vi "Get JSON Data.vi"(7 "Panel Origin":T1, 8 "error in (no error)":errorcluster, 9 "Force Get All Data":bool, 10 "VI Reference":refnum<vi>, 11 "Select In":refnum<class "Select.lvclass">) -> (0 "error out":errorcluster, 2 "JSON string":string, 3 "Select Out":refnum<class "Select.lvclass">)   [LabVIEW 2015, in "Front Panel Publisher.lvlib" / "Select.lvclass"]
uses:
  Select.lvclass
  <vilib>/Utility/miscctls.llb/LVPointTypeDef.ctl
  Text_class/Text.lvclass
  Control_class/Control.lvclass
  Object_class/Object.lvclass
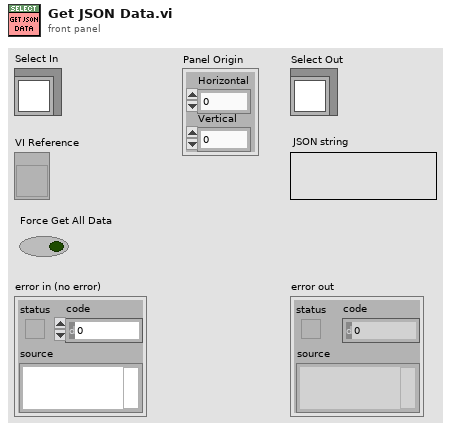
[diagram p1: front panel]
types:
  T1 = typedef "LVPointTypeDef.ctl" = cluster{"Horizontal":i16, "Vertical":i16}
  T2 = typedef "Front Panel Publisher.lvlib/Object.lvclass/Attributes.ctl" = cluster{"UID":i32, "Type":string, "Coordinates":T3, "Reference":refnum<vi>}
  T3 = typedef "Front Panel Publisher.lvlib/Object.lvclass/Coordinates.ctl" = cluster{"Left":i32, "Top":i32, "Height":u32, "Width":u32}
  T4 = typedef "Front Panel Publisher.lvlib/Control.lvclass/Attributes.ctl" = cluster{"Description":string, "Indicator":bool, "Default Value":variant, "Control Index":i32, "Label":refnum<class "Text.lvclass">, "Caption":refnum<class "Text.lvclass">, "Image b64":string, "Use Picture":bool, "Value Only":bool}
  T5 = typedef "Front Panel Publisher.lvlib/Select.lvclass/Attributes.ctl" = cluster{"Ring Image Variable Name":string}
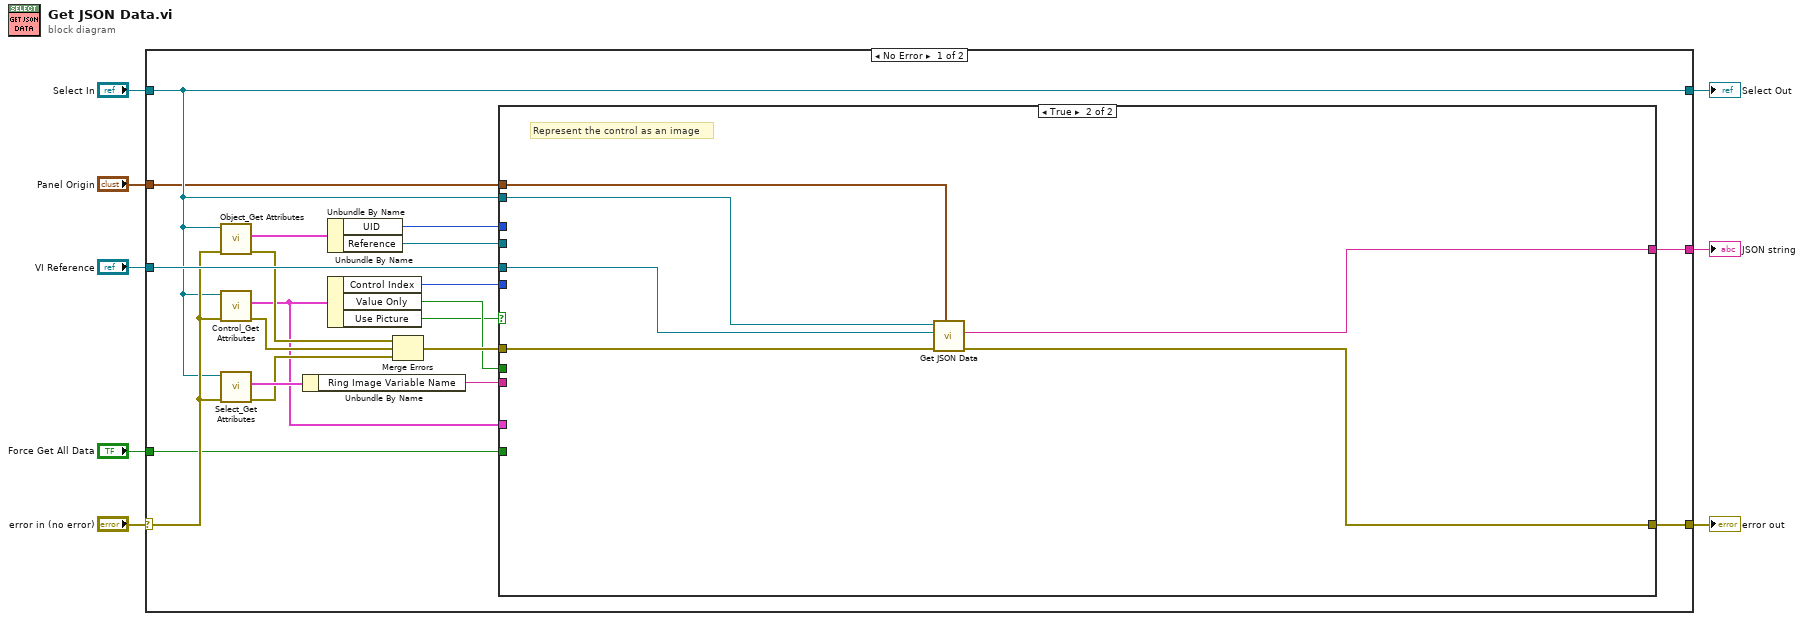
[diagram p0: block diagram]
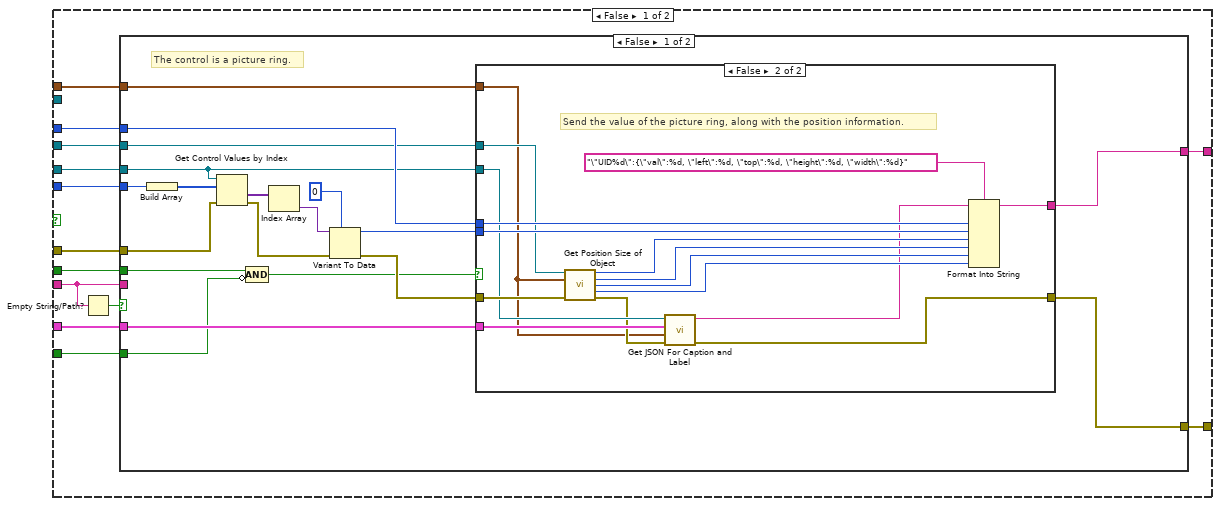
[diagram p2: hidden frame]
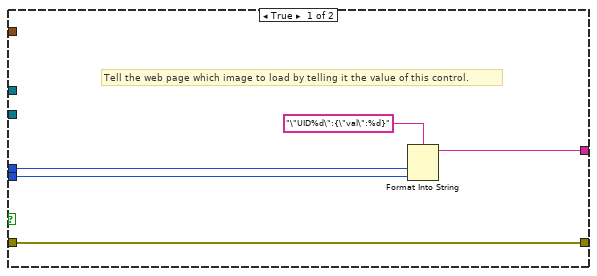
[diagram p3: hidden frame]
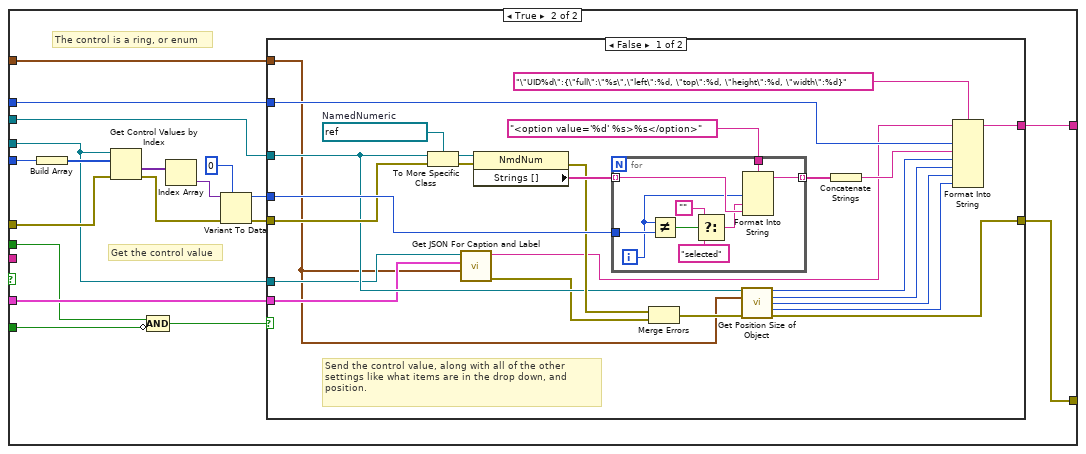
[diagram p4: hidden frame]
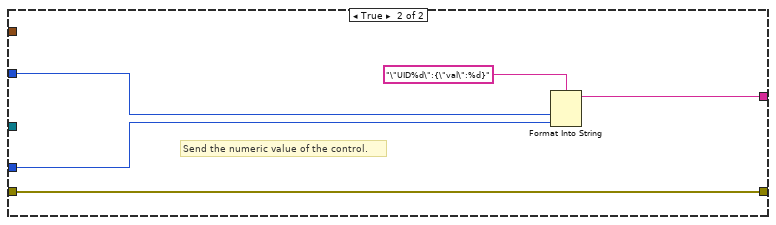
[diagram p5: hidden frame]
diagram:
  n1 = case shown="No Error" "error in (no error)" {
    selector: "error in (no error)" -> [w19 w147]
    tunnel: [w27 w147] -> w7
    tunnel: [w12 w146] -> w5
    tunnel: "Select In" -> [w12 w146]
    tunnel: "VI Reference" -> [w25 _]
    tunnel: [w24 _] -> w3
    tunnel: "Force Get All Data" -> [w10 _]
    tunnel: "Panel Origin" -> [w9 _]
    frame No Error {
      n2 = call "Object_Get Attributes.vi"("error in (no error)"=w19, "Object In"=w12) -> ("error out"=w17:errorcluster, "Data"=w23:T2)  [unwired: 6 in, 2 out]
      n3 = call "Control_Get Attributes.vi"("error in (no error)"=w19, "Control In"=w12) -> ("error out"=w28:errorcluster, "Data"=w11:T4)  [unwired: 6 in, 2 out]
      n4 = call "Select_Get Attributes.vi"("error in (no error)"=w19, "Select In"=w12) -> ("error out"=w16:errorcluster, "Data"=w20:T5)  [unwired: 6 in, 2 out]
      n5 = Unbundle By Name(w20) -> ("Ring Image Variable Name"=w15:string)
      n6 = Unbundle By Name(w23) -> ("UID"=w22:i32, "Reference"=w21:refnum<vi>)
      n7 = Unbundle By Name(w11) -> ("Control Index"=w26:i32, "Value Only"=w14:bool, "Use Picture"=w13:bool)
      n8 = Merge Errors(w17, w28, w16) -> (w18:errorcluster)
      n9 = case shown="True" w13 {
        tunnel: [w41 w142] -> w27
        tunnel: w26 -> [w40 _]
        tunnel: w25 -> [w39 w144]
        tunnel: [w38 w141] -> w24
        tunnel: w22 -> [w37 _]
        tunnel: w21 -> [w36 _]
        tunnel: w18 -> [w35 w143]
        tunnel: w15 -> [w33 _]
        tunnel: w14 -> [w32 _]
        tunnel: w12 -> [_ w145]
        tunnel: w11 -> [w31 _]
        tunnel: w10 -> [w30 _]
        tunnel: w9 -> [w29 w140]
        frame False {
          n10 = Empty String/Path?(string/path=w33) -> (empty?=w34:bool)
          n11 = case shown="False" w34 {
            tunnel: [w48 w100] -> w41
            tunnel: w40 -> [w55 w99]
            tunnel: w39 -> [w46 w87]
            tunnel: [w53 w98] -> w38
            tunnel: w37 -> [w54 w97]
            tunnel: w36 -> [w50 w88]
            tunnel: w35 -> [w52 w96]
            tunnel: w33 -> [_ _]
            tunnel: w32 -> [w44 w84]
            tunnel: w31 -> [w47 w86]
            tunnel: w30 -> [w45 w85]
            tunnel: w29 -> [w42 w82]
            frame False {
              # "The control is a picture ring."
              n12 = Build Array(w55) -> (w59:i32[])
              n13 = Get Control Values by Index(0:w46, 1:w59, 3:w52) -> (10:w58:variant[], 11:w60:errorcluster)
              n14 = Compound Arithmetic op=AND(w44, invert w45) -> (w43:bool)
              n15 = Index Array(array=w58) -> (element=w57:variant)  [unwired: 1 in]
              n16 = Variant To Data(error in=w60, type=0, Variant=w57) -> (data=w51:i32, error out=w49:errorcluster)
              n17 = case shown="False" w43 {
                tunnel: w54 -> [w65 w81]
                tunnel: [w64 w80] -> w53
                tunnel: w51 -> [w63 w79]
                tunnel: w50 -> [_ w77]
                tunnel: w49 -> [w61 w72]
                tunnel: [w61 w67] -> w48
                tunnel: w47 -> [_ w71]
                tunnel: w46 -> [_ w70]
                tunnel: w42 -> [_ w66]
                frame True {
                  # "Tell the web page which image to load by telling it the value of this control."
                  n18 = Format Into String(format string="\"UID%d\":{\"val\":%d}", w65, w63) -> (resulting string=w64:string)  [unwired: 2 in, 1 out]
                }
                frame False {
                  # "Send the value of the picture ring, along with the position information."
                  n19 = call "Get Position Size of Object.vi"("GObject in"=w77, "Panel Origin"=w66, "error in (no error)"=w72) -> ("Left"=w76:i32, "Top"=w75:i32, "Height"=w74:u32, "Width"=w73:u32, "error out"=w68:errorcluster)  [unwired: 8 in]
                  n20 = call "Get JSON For Caption and Label.vi"("error in (no error)"=w68, "Panel Origin"=w66, "Data"=w71, "VI in"=w70) -> ("error out"=w67:errorcluster, "JSON"=w69:string)  [unwired: 6 in]
                  n21 = Format Into String(format string="\"UID%d\":{\"val\":%d, \"left\":%d, \"top\":%d, \"height\":%d, \"width\":%d}", initial string=w69, w81, w79, w76, w75, w74, w73) -> (resulting string=w80:string)  [unwired: 1 in, 1 out]
                }
              }
            }
            frame True {
              # "Get the control value"
              # "The control is a ring, or enum"
              n22 = Build Array(w99) -> (w93:i32[])
              n23 = Get Control Values by Index(0:w87, 1:w93, 3:w96) -> (10:w92:variant[], 11:w95:errorcluster)
              n24 = Compound Arithmetic op=AND(w84, invert w85) -> (w83:bool)
              n25 = Index Array(array=w92) -> (element=w91:variant)  [unwired: 1 in]
              n26 = Variant To Data(error in=w95, type=0, Variant=w91) -> (data=w89:i32, error out=w94:errorcluster)
              n27 = case shown="False" w83 {
                tunnel: [w112 w135] -> w100
                tunnel: [w117 w139] -> w98
                tunnel: w97 -> [w116 w138]
                tunnel: w94 -> [w114 w135]
                tunnel: w89 -> [w115 w136]
                tunnel: w88 -> [w107 _]
                tunnel: w87 -> [w106 _]
                tunnel: w86 -> [w105 _]
                tunnel: w82 -> [w101 _]
                frame False {
                  w123 = refnum<vi> refnum  # NamedNumeric
                  # "Send the control value, along with all of the other settings like what items are in the drop down, and position."
                  n28 = To More Specific Class(target class=w123, reference=w107, error in=w114) -> (specific class reference=w121:refnum<vi>, error out=w122:errorcluster)
                  n29 = call "Get JSON For Caption and Label.vi"("Panel Origin"=w101, "Data"=w105, "VI in"=w106) -> ("error out"=w102:errorcluster, "JSON"=w104:string)  [unwired: 7 in]
                  n30 = property class="NmdNum"(reference=w121, error in=w122) -> (error out=w113:errorcluster, "Strings []"=w120:string[])  [unwired: 1 out]
                  n31 = for {
                    tunnel: w120 -> [w133] mode=indexing
                    tunnel: "<option value='%d' %s>%s</option>" -> [w134]
                    tunnel: w115 -> [w131]
                    tunnel: [w129] -> w118 mode=indexing
                    i -> [w128]
                    n32 = Not Equal?(x=w128, y=w131) -> (x != y?=w132:bool)
                    n33 = Select(t="", s=w132, f="selected") -> (s? t:f=w130:string)
                    n34 = Format Into String(format string=w134, w128, w130, w133) -> (resulting string=w129:string)  [unwired: 2 in, 1 out]
                  }
                  n35 = Merge Errors(w113, w102) -> (w103:errorcluster)
                  n36 = call "Get Position Size of Object.vi"("GObject in"=w107, "Panel Origin"=w101, "error in (no error)"=w103) -> ("Left"=w111:i32, "Top"=w110:i32, "Height"=w109:u32, "Width"=w108:u32, "error out"=w112:errorcluster)  [unwired: 8 in]
                  n37 = Concatenate Strings(w118) -> (w125:string)
                  n38 = Format Into String(format string="\"UID%d\":{\"full\":\"%s\",\"left\":%d, \"top\":%d, \"height\":%d, \"width\":%d}", initial string=w104, w116, w125, w111, w110, w109, w108) -> (resulting string=w117:string)  [unwired: 1 in, 1 out]
                }
                frame True {
                  # "Send the numeric value of the control."
                  n39 = Format Into String(format string="\"UID%d\":{\"val\":%d}", w138, w136) -> (resulting string=w139:string)  [unwired: 2 in, 1 out]
                }
              }
            }
          }
        }
        frame True {
          # "Represent the control as an image"
          n40 = call-parent "Get JSON Data.vi"("Panel Origin"=w140, "error in (no error)"=w143, "VI Reference"=w144, "Control In"=w145) -> ("error out"=w142:errorcluster, "JSON string"=w141:string)  [unwired: 5 in, 1 out]
        }
      }
    }
    frame Error {
    }
  }
  "error out" <- w7
  "Select Out" <- w5
  "JSON string" <- w3
